vi "Read UserEventCommand.vi"(8 "error in (no error)":errorcluster caption="entrée d'erreur (pas d'erreur)", 11 "Control en entrée":refnum<class "Control.lvclass">) -> (0 "error out":errorcluster caption="sortie d'erreur", 2 "UserEventCommand":refnum<user-event>, 3 "Control en sortie":refnum<class "Control.lvclass">)   [LabVIEW 2015, in "Control.lvclass"]
uses:
  Control.lvclass
  Control.lvclass/Control.ctl
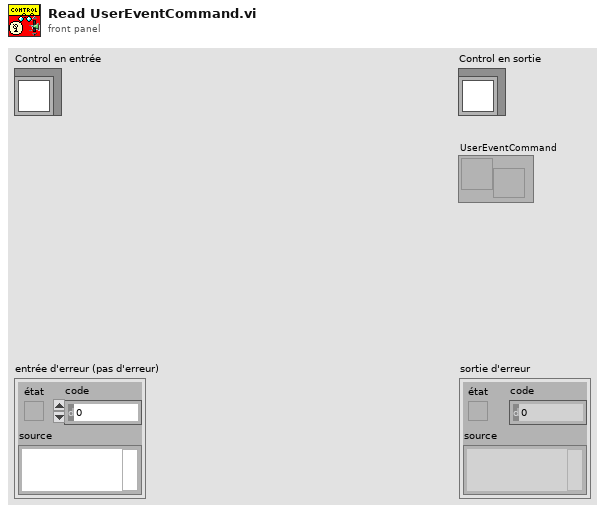
[diagram p1: front panel]
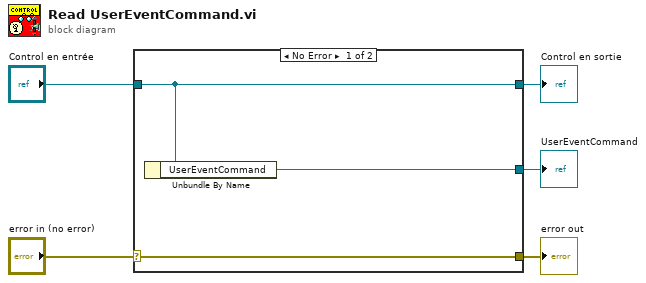
[diagram p0: block diagram]
diagram:
  n1 = case shown="No Error" "error in (no error)" {
    selector: "error in (no error)" -> [w8 w9]
    tunnel: [w8 w9] -> w4
    tunnel: [w7 w10] -> w2
    tunnel: "Control en entrée" -> [w7 w10]
    tunnel: [w6 _] -> w1
    frame No Error {
      n2 = Unbundle By Name(w7) -> ("UserEventCommand"=w6:refnum<user-event>)
    }
    frame Error {
    }
  }
  "error out" <- w4
  "Control en sortie" <- w2
  "UserEventCommand" <- w1
